vi "USB_kernal_server.vi"(0 "Board type":T2=enum."Local ADAM", 1 "Sync Mode?":bool, 2 "Client Time":dbl, 5 "No of samples+extra":i32=128 min=0 step=1, 7 "Trigger mode":T1, 9 "output polarity":u16(ring)=1 items=["do not change", "positive", "negative"], 11 "Ch & spans":T3[](array[typedef]) {"low limit (-10V)" format="%.3f"; "high limit (10V)" format="%.3f"}, 12 "Actual Sampling rate (Hz)":dbl=1000.0 format="%.2f", 13 "Local Client?":bool, 14 "Current Block No":i32) -> (4 "I16 data":i16[][](array[numeric]), 6 "Block Timings":T4={"Started"=0.0, "Ended"=0.0, "Analogue Frequency Hz"=1000.0} {"Analogue Frequency Hz" format="%.2f"}, 10 "group channel settings":T5(array[cluster]) {"scale offset" format="%.2f"; "scale multiplier" format="%.2f"; "gain" format="%.2f"; "range" format="%.2f"; "lower input limits" format="%.2f"; "upper input limits" format="%.2f"}, 15 "error out":errorcluster)   [LabVIEW 2015]
uses:
  Controls/Block_start_and_end.ctl
  Controls/Ch_and_Spans.ctl
  Controls/Board_Types.ctl
  Controls/Trigger_Mode.ctl
  PWA/PWAtasksGLOBAL.vi
  <vilib>/_DAQmxBase/Internals/DAQmxBase Create Channel (AI-Voltage-Basic).vi
  <vilib>/_DAQmxBase/Internals/DAQmxBase Timing (Sample Clock).vi
  Globals/Meas_global.vi
  Globals/LDA_meas_global_1.vi
  <vilib>/_DAQmxBase/Internals/DAQmxBase Read (Analog 2D DBL NChan NSamp).vi
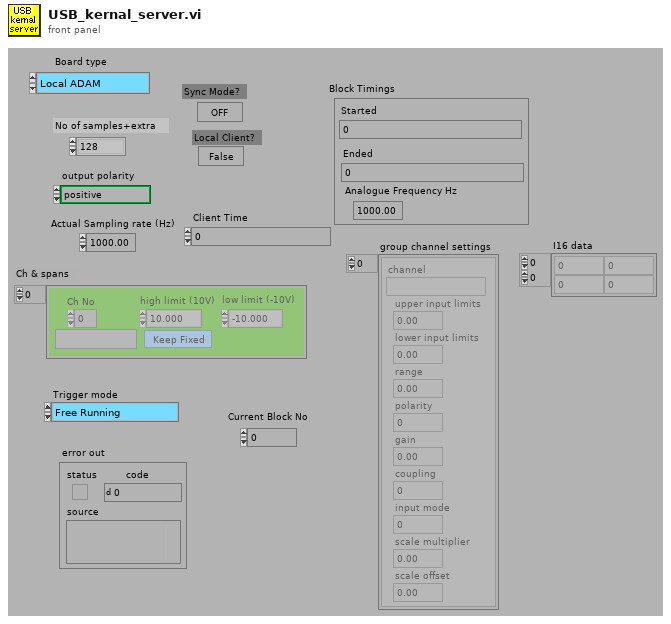
[diagram p1: front panel]
types:
  T1 = typedef "Trigger_Mode.ctl" = enum16{"Free Running", "Start on Trigger", "Trigger Every Block", "Trigger Every Sample"}
  T2 = typedef "Board_Types.ctl" = enum16{"Simulate", "Local ADAM", "Server ADAM", "NI-DAQmx", "NI-DAQmxBase", "ADC488", "DT LV-link"}
  T3 = typedef "Ch_and_Spans.ctl" = cluster{"high limit (10V)":sgl, "low limit (-10V)":sgl, "Ch No":i16, "Var name":string, "Use Latest Calib":bool}
  T4 = typedef "Block_start_and_end.ctl" = cluster{"Started":dbl, "Ended":dbl, "Analogue Frequency Hz":dbl}
  T5 = cluster{"channel":string, "upper input limits":sgl, "lower input limits":sgl, "range":sgl, "polarity":u16, "gain":sgl, "coupling":u16, "input mode":u16, "scale multiplier":dbl, "scale offset":dbl}[]
  T6 = typedef "BSA_info_Cluster.ctl" = cluster{"GPIB Address":string, "No of Check Bytes":i32, "Extra Info":string, "COLOUR":u32, "Wavelength (nm)":dbl}
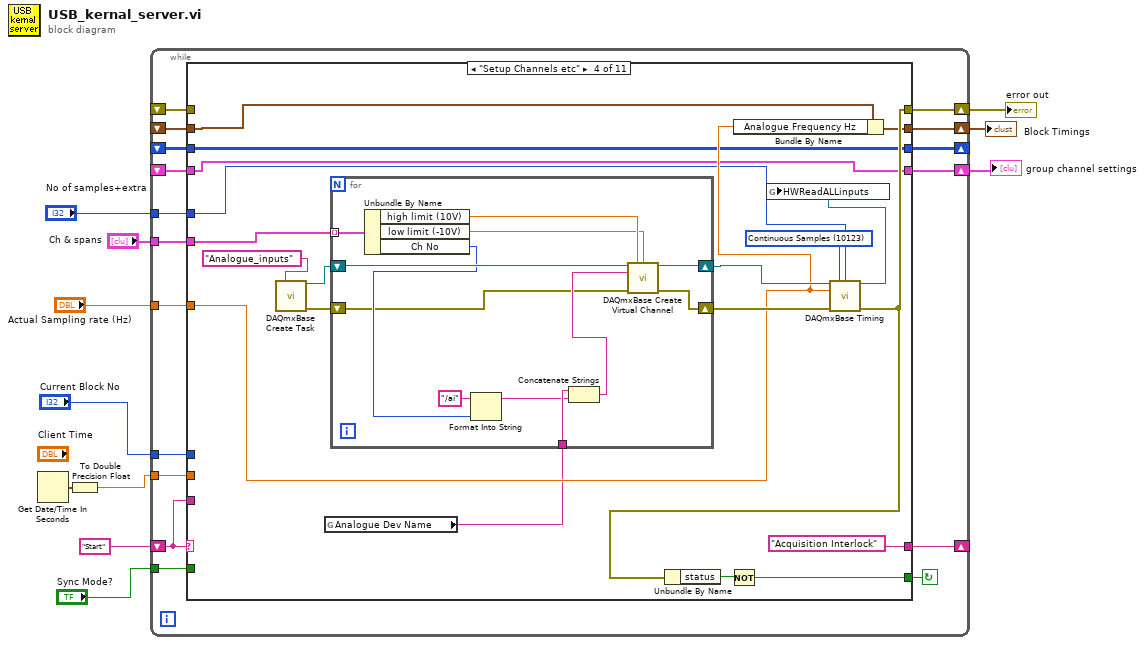
[diagram p0: block diagram]
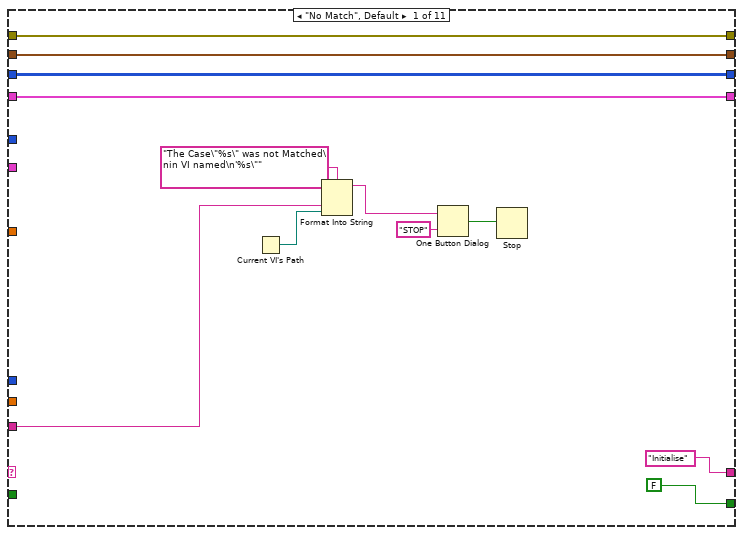
[diagram p2: hidden frame]
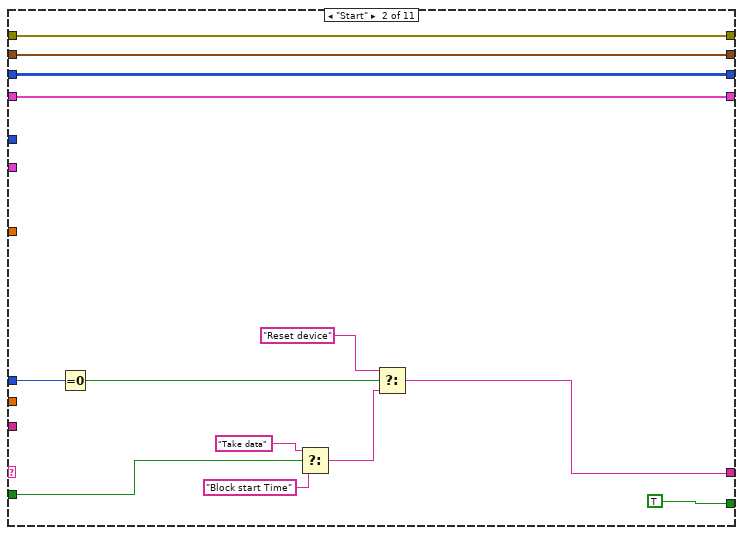
[diagram p3: hidden frame]
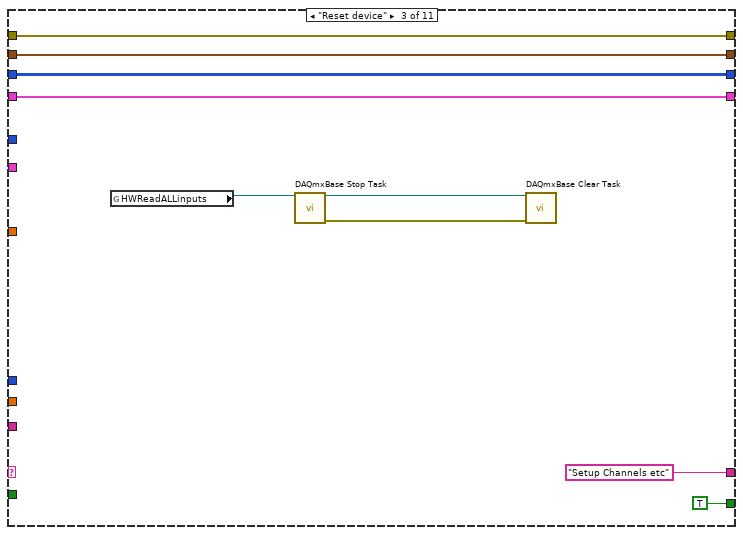
[diagram p4: hidden frame]
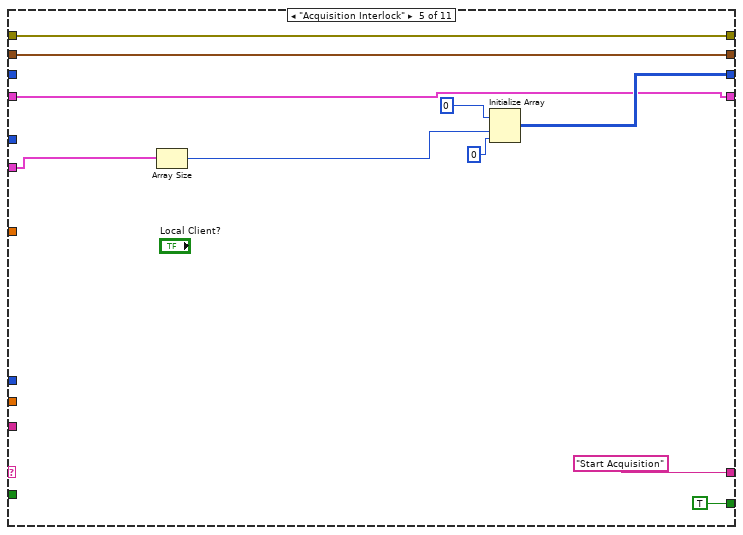
[diagram p5: hidden frame]
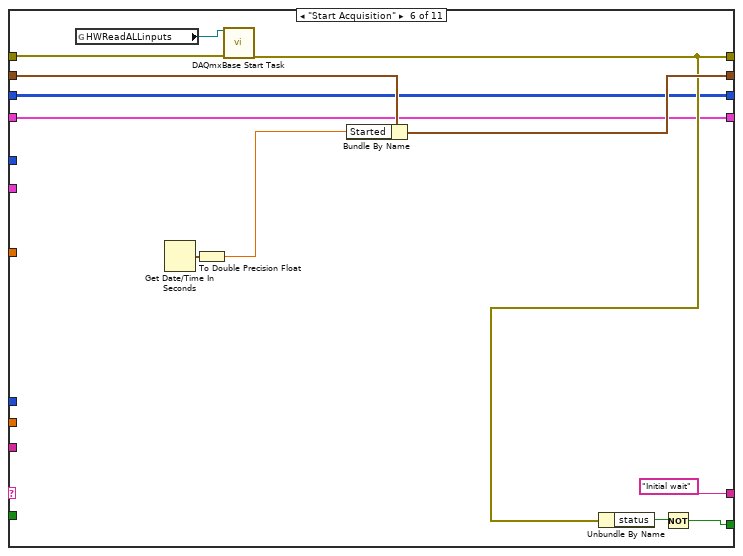
[diagram p6: hidden frame]
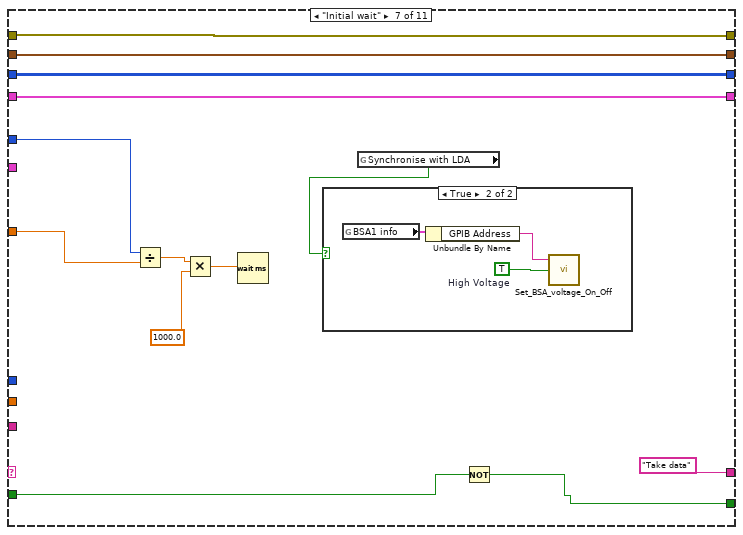
[diagram p7: hidden frame]
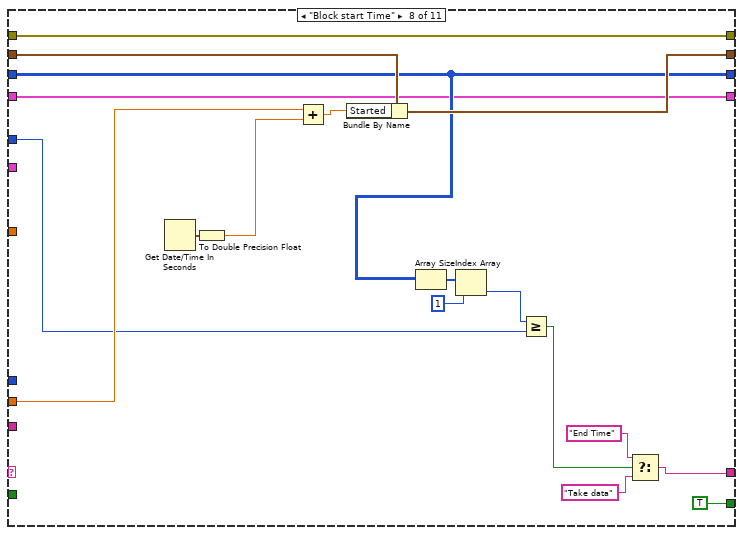
[diagram p9: hidden frame]
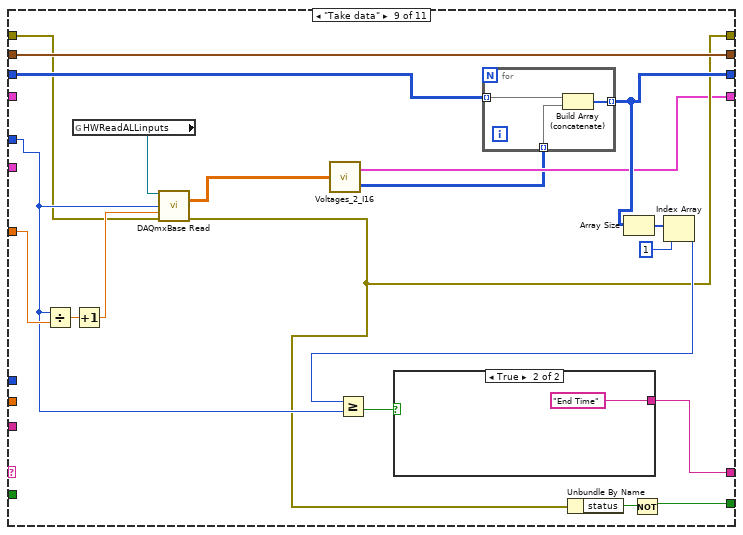
[diagram p10: hidden frame]
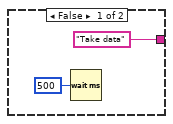
[diagram p11: hidden frame]
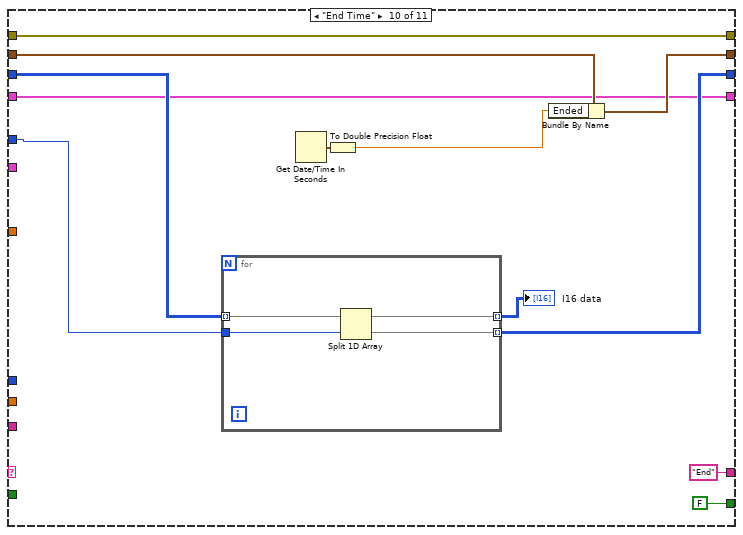
[diagram p12: hidden frame]
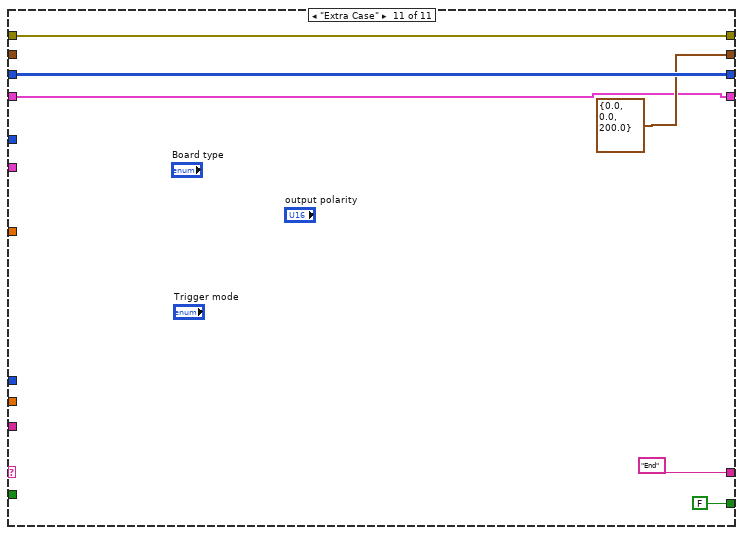
[diagram p13: hidden frame]
diagram:
  n1 = Get Date/Time In Seconds() -> (seconds since 1Jan1904=w10:timestamp)
  n2 = To Double Precision Float(number=w10) -> (double precision float=w1:dbl)
  n3 = while {
    shift-left: "Start" -> [w26]
    shift-right: [w27] -> _
    shift-right: [w25] -> w9
    shift-left: _ -> [w24]
    shift-right: [w23] -> w8
    shift-left: _ -> [w22]
    tunnel: w1 -> [w21]
    tunnel: "Actual Sampling rate (Hz)" -> [w20]
    tunnel: "No of samples+extra" -> [w19]
    shift-right: [w16] -> _
    shift-left: _ -> [w17]
    tunnel: "Current Block No" -> [w18]
    tunnel: "Ch & spans" -> [w15]
    shift-right: [w14] -> w3
    shift-left: _ -> [w13]
    tunnel: "Sync Mode?" -> [w12]
    stop <- w28 continue-if-true
    n4 = case shown="\"Setup Channels etc\"" w26 {
      tunnel: [FALSE TRUE TRUE w73 TRUE w109 w117 TRUE w158 FALSE FALSE] -> w28
      tunnel: ["Initialise" w46 "Setup Channels etc" "Acquisition Interlock" "Start Acquisition" "Initial wait" "Take data" w134 w161 "End" ("f") "End"] -> w27
      tunnel: w26 -> [w35 _ _ _ _ _ _ _ _ _ _]
      tunnel: [w32 w52 w58 w75 w102 w108 w126 w143 w153 w187 w196] -> w25
      tunnel: w24 -> [w32 w52 w58 _ w102 w111 w126 w143 w154 w187 w196]
      tunnel: [w31 w51 w61 w71 w100 w112 w125 w147 w169 w183 T4 {"Started"=0.0, "Ended"=0.0, "Analogue Frequency Hz"=200.0} ("Block Timings")] -> w23
      tunnel: w22 -> [w31 w51 w61 w72 w100 w113 w125 w148 w169 w184 _]
      tunnel: w21 -> [_ _ _ _ _ _ _ w145 _ _ _]
      tunnel: w20 -> [_ _ _ w70 _ _ w123 _ w168 _ _]
      tunnel: w19 -> [_ _ _ w69 _ _ w124 w137 w156 w182 _]
      tunnel: w18 -> [_ w49 _ _ _ _ _ _ _ _ _]
      tunnel: w17 -> [w30 w50 w57 w67 _ w107 w127 w139 w166 w181 w194]
      tunnel: [w30 w50 w57 w67 w95 w107 w127 w139 w165 w179 w194] -> w16
      tunnel: w15 -> [_ _ _ w68 w98 _ _ _ _ _ _]
      tunnel: [w29 w45 w55 w66 w94 w106 w119 w132 w152 w177 w192] -> w14
      tunnel: w13 -> [w29 w45 w55 w66 w94 w106 w119 w132 _ w177 w192]
      tunnel: w12 -> [_ w44 _ _ _ _ w116 _ _ _ _]
      frame "No Match", Default {
        n5 = Current VI's Path() -> (path=w34:path)
        n6 = Format Into String(format string="The Case\"%s\" was not Matched\nin VI named\n'%s\"" ("Format String"), w35, w34) -> (resulting string=w38:string)  [unwired: 2 in, 1 out]
        n7 = One Button Dialog(message=w38, button name ("OK")="STOP") -> (true=w36:bool)
        n8 = Stop(stop? (T)=w36) -> ()
      }
      frame "Start" {
        n9 = Equal To 0?(x=w49) -> (x = 0?=w47:bool)
        n10 = Select(t="Take data", s=w44, f="Block start Time") -> (s? t:f=w43:string)
        n11 = Select(t="Reset device", s=w47, f=w43) -> (s? t:f=w46:string)
      }
      frame "Reset device" {
        n12 = global read "PWAtasksGLOBAL.vi" "HWReadALLinputs"() -> (w54:refnum<k21>)
        n13 = call <vilib>:"DAQmxBase Stop Task.vi"("task/channels in"=w54) -> ("task out"=w60:refnum<k21>, "error out"=w59:errorcluster)  [unwired: 13 in]
        n14 = call <vilib>:"DAQmxBase Clear Task.vi"("task in"=w60, "error in"=w59) -> ()  [unwired: 13 in, 1 out]
      }
      frame "Setup Channels etc" {
        w78 = 10123 items=["Finite Samples"=10178, "Continuous Samples"=10123, "Hardware Timed Single Point"=12522] ("sample mode")
        n15 = call <vilib>:"DAQmxBase Create Task.vi"("new task name"="Analogue_inputs") -> ("task out"=w76:refnum<k21>, "error out"=w79:errorcluster)  [unwired: 13 in]
        n16 = global read "PWAtasksGLOBAL.vi" "Analogue Dev Name"() -> (w63:string)
        n17 = for {
          tunnel: w68 -> [w93] mode=indexing
          shift-right: [w89] -> w77
          shift-left: w76 -> [w90]
          shift-right: [w88] -> w80
          shift-left: w79 -> [w82]
          tunnel: w63 -> [w87]
          n18 = Unbundle By Name(w93) -> ("high limit (10V)"=w92:sgl, "low limit (-10V)"=w91:sgl, "Ch No"=w85:i16)
          n19 = Format Into String(initial string="/ai", w85) -> (resulting string=w83:string)  [unwired: 2 in, 1 out]
          n20 = Concatenate Strings(w87, w83) -> (w86:string)
          n21 = call-poly <vilib>:"DAQmxBase Create Virtual Channel.vi"("task in"=w90, "maximum value"=w92, "minimum value"=w91, "physical channels"=w86, "error in"=w82) -> ("task out"=w89:refnum<k21>, "error out"=w88:errorcluster)  [unwired: 9 in]
        }
        n22 = Bundle By Name(cluster=w72, "Analogue Frequency Hz"=w70) -> (w71:T4)
        n23 = call-poly <vilib>:"DAQmxBase Timing.vi"("task/channels in"=w77, "sample mode"=w78, "samples per channel"=w69, "rate"=w70, "error in"=w80) -> ("task out"=w64:refnum<k21>, "error out"=w75:errorcluster)  [unwired: 9 in]
        n24 = Unbundle By Name(w75) -> ("status"=w74:bool)
        n25 = Not(x=w74) -> (.not. x?=w73:bool)
        n26 = global write "PWAtasksGLOBAL.vi" "HWReadALLinputs"(w64) -> ()
      }
      frame "Acquisition Interlock" {
        n27 = Array Size(array=w98) -> (size(s)=w97:i32)
        n28 = Initialize Array(i16 0, w97, 0 ("dimension size")) -> (w95:i16[][])
      }
      frame "Start Acquisition" {
        n29 = global read "PWAtasksGLOBAL.vi" "HWReadALLinputs"() -> (w105:refnum<k21>)
        n30 = Get Date/Time In Seconds() -> (seconds since 1Jan1904=w114:timestamp)
        n31 = To Double Precision Float(number=w114) -> (double precision float=w104:dbl)
        n32 = call <vilib>:"DAQmxBase Start Task.vi"("task/channels in"=w105, "error in"=w111) -> ("error out"=w108:errorcluster)  [unwired: 12 in, 1 out]
        n33 = Bundle By Name(cluster=w113, "Started"=w104) -> (w112:T4)
        n34 = Unbundle By Name(w108) -> ("status"=w110:bool)
        n35 = Not(x=w110) -> (.not. x?=w109:bool)
      }
      frame "Initial wait" {
        n36 = Divide(x=w124, y=w123) -> (x/y=w122:dbl)
        n37 = Multiply(x=w122, y=1000.0) -> (x*y=w120:dbl)
        n38 = Wait (ms)(milliseconds to wait=w120) -> ()  [unwired: 1 out]
        n39 = global read "Meas_global.vi" "Synchronise with LDA"() -> (w118:bool)
        n40 = case shown="True" w118 {
          frame False {
          }
          frame True {
            w129 = TRUE  # High Voltage
            n41 = global read "LDA_meas_global_1.vi" "BSA1 info"() -> (w130:T6)
            n42 = Unbundle By Name(w130) -> ("GPIB Address"=w131:string)
            n43 = call "Set_BSA_voltage_On_Off.vi"("GPIB address"=w131, "High Voltage"=w129) -> ()  [unwired: 5 in, 1 out]
          }
        }
        n44 = Not(x=w116) -> (.not. x?=w117:bool)
      }
      frame "Block start Time" {
        n45 = Get Date/Time In Seconds() -> (seconds since 1Jan1904=w149:timestamp)
        n46 = To Double Precision Float(number=w149) -> (double precision float=w146:dbl)
        n47 = Add(x=w145, y=w146) -> (x+y=w144:dbl)
        n48 = Bundle By Name(cluster=w148, "Started"=w144) -> (w147:T4)
        n49 = Array Size(array=w139) -> (size(s)=w141:i32[])
        n50 = Index Array(array=w141, index=1) -> (element=w138:i32)
        n51 = Greater Or Equal?(x=w138, y=w137) -> (x >= y?=w136:bool)
        n52 = Select(t="End Time", s=w136, f="Take data") -> (s? t:f=w134:string)
      }
      frame "Take data" {
        n53 = Divide(x=w156, y=w168) -> (x/y=w167:dbl)
        n54 = global read "PWAtasksGLOBAL.vi" "HWReadALLinputs"() -> (w157:refnum<k21>)
        n55 = Increment(x=w167) -> (x+1=w155:dbl)
        n56 = call-poly <vilib>:"DAQmxBase Read.vi"("task/channels in"=w157, "number of samples per channel"=w156, "timeout"=w155, "error in"=w154) -> ("data"=w150:dbl[][], "error out"=w153:errorcluster)  [unwired: 9 in, 1 out]
        n57 = call "Voltages_2_I16.vi"("Voltages"=w150) -> ("Group Channel Settings"=w152:T5, "I16 data"=w151:i16[][])
        n58 = for {
          tunnel: w151 -> [w175] mode=indexing
          tunnel: w166 -> [w174] mode=indexing
          tunnel: [w173] -> w165 mode=indexing
          n59 = Build Array (concatenate)(w174, w175) -> (w173:i16[])
        }
        n60 = Unbundle By Name(w153) -> ("status"=w159:bool)
        n61 = Array Size(array=w165) -> (size(s)=w164:i32[])
        n62 = Not(x=w159) -> (.not. x?=w158:bool)
        n63 = Index Array(array=w164, index=1) -> (element=w162:i32)
        n64 = Greater Or Equal?(x=w162, y=w156) -> (x >= y?=w160:bool)
        n65 = case shown="True" w160 {
          tunnel: ["Take data" "End Time"] -> w161
          frame False {
            n66 = Wait (ms)(milliseconds to wait=u32 500) -> ()  [unwired: 1 out]
          }
          frame True {
          }
        }
      }
      frame "End Time" {
        n67 = for {
          tunnel: w181 -> [w191] mode=indexing
          tunnel: w182 -> [w190]
          tunnel: [w189] -> w178 mode=indexing
          tunnel: [w188] -> w179 mode=indexing
          n68 = Split 1D Array(array=w191, index=w190) -> (first subarray=w189:i16[], second subarray=w188:i16[])
        }
        "I16 data" <- w178
        n69 = Get Date/Time In Seconds() -> (seconds since 1Jan1904=w185:timestamp)
        n70 = To Double Precision Float(number=w185) -> (double precision float=w176:dbl)
        n71 = Bundle By Name(cluster=w184, "Ended"=w176) -> (w183:T4)
      }
      frame "Extra Case" {
      }
    }
  }
  "error out" <- w9
  "Block Timings" <- w8
  "group channel settings" <- w3
